vi "LinkFixToSerialNumber.vi"(0 "class data in":refnum<class "CMESAPI.lvclass">, 5 "serialNumber":string, 7 "equipment":string, 9 "WorkorderNumber":string, 11 "error in (no error)":errorcluster) -> (4 "class data out":refnum<class "CMESAPI.lvclass">, 6 "resulting string":string, 15 "error out":errorcluster)   [LabVIEW 2020, in "Salcomp-MES.lvlib" / "CMESAPI.lvclass"]
uses:
  CMESAPI.lvclass
  CMESAPI.lvclass/CMESAPI.ctl
  E:/Git/Libraries/develop/CME-API/CMESAPI_Fw4.0_1.9.2/CMESAPI.dll
  CMESAPI_Fw4.0_1.9.2/CMESAPI.dll
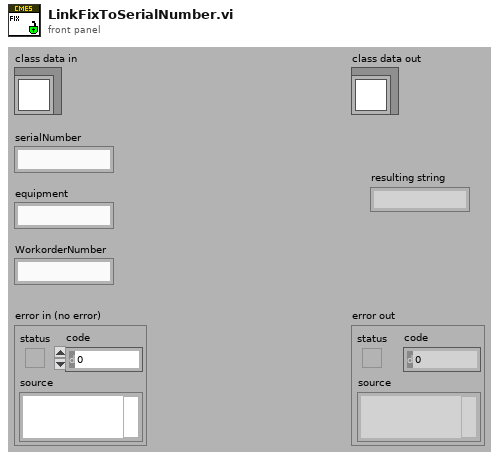
[diagram p1: front panel]
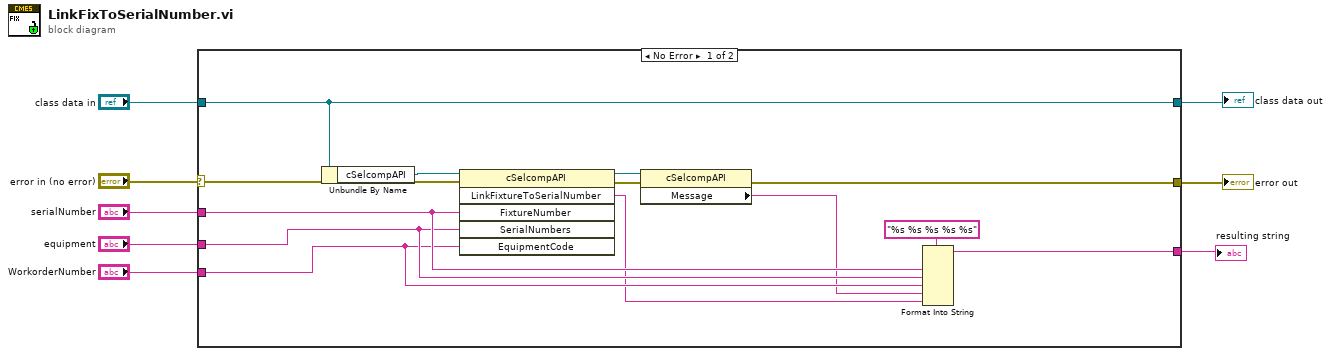
[diagram p0: block diagram]
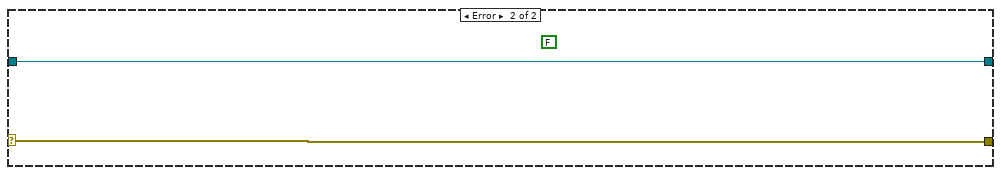
[diagram p2: hidden frame]
diagram:
  n1 = case shown="No Error" "error in (no error)" {
    selector: "error in (no error)" -> [w19 w23]
    tunnel: [w15 w23] -> w7
    tunnel: "class data in" -> [w21 w22]
    tunnel: [w21 w22] -> w5
    tunnel: "WorkorderNumber" -> [w12 _]
    tunnel: "equipment" -> [w13 _]
    tunnel: "serialNumber" -> [w14 _]
    tunnel: [w9 _] -> w1
    frame No Error {
      n2 = Unbundle By Name(w21) -> ("cSelcompAPI"=w20:refnum<k24>)
      n3 = invoke on="Invoke Node" class="cSelcompAPI" method="LinkFixtureToSerialNumber"(reference=w20, error in=w19, "FixtureNumber"=w14, "SerialNumbers"=w13, "EquipmentCode"=w12) -> (reference out=w18:refnum<k24>, error out=w17:errorcluster, "LinkFixtureToSerialNumber"=w10:string)  [unwired: 1 in, 3 out]
      n4 = property class="cSelcompAPI"(reference=w18, error in=w17) -> (error out=w15:errorcluster, "Message"=w11:string)  [unwired: 1 out]
      n5 = Format Into String(format string="%s %s %s %s %s", w14, w13, w12, w11, w10) -> (resulting string=w9:string)  [unwired: 2 in, 1 out]
    }
    frame Error {
      (unwired) FALSE ("CheckRouteForSerialNumber")
    }
  }
  "error out" <- w7
  "class data out" <- w5
  "resulting string" <- w1
